vi "SetupDMA.vi"(0 "blocks":u32=1, 2 "pixel":u32=2400, 3 "nos":u32=1) -> (1 "Data Values":u16[][](graph))   [LabVIEW 2015]
uses:
  ESLSCDLL.dll
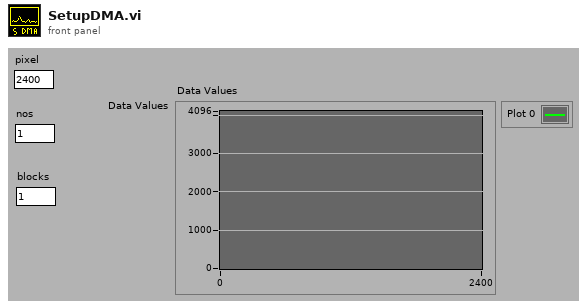
[diagram p1: front panel]
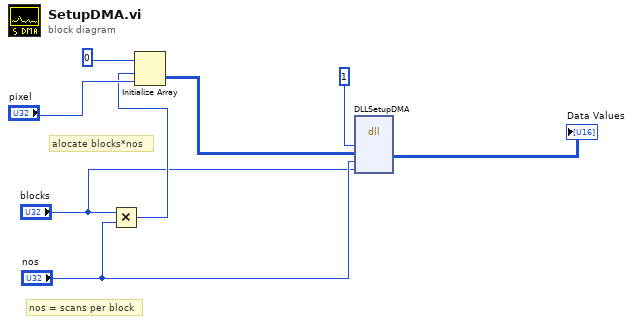
[diagram p0: block diagram]
diagram:
  # "alocate blocks*nos"
  # "nos = scans per block"
  n1 = Multiply(x="blocks", y="nos") -> (x*y=w2:u32)
  n2 = Initialize Array(u16 0, w2, "pixel") -> (w6:u16[][])
  n3 = dll-call lib="C:/ENTW/PCIE/64bit/lv64/1cam/board.vis/ESLSCDLL.dll" fn="DLLSetupDMA" ("lwlscdll.dll:DLLReadFFLoop")("drv"=u32 1, "dioden"=w6, "nos"="nos", "blocks"="blocks") -> ("dioden"=→"Data Values":u16[][])  [unwired: 7 in, 2 out]
